vi "Begin.vi"(8 "error in (no error)":errorcluster, 11 "Two Drivers in":refnum<class "Two Drivers.lvclass">) -> (0 "error out":errorcluster, 3 "Two Drivers out":refnum<class "Two Drivers.lvclass">)   [LabVIEW 2018, in "Joysticks.lvlib" / "Two Drivers.lvclass"]
doc: "This VI is used to open the joystick control references."
uses:
  Two Drivers.lvclass
  <vilib>/Rock Robotics/WPI/Joystick/WPI_JoystickDeviceEnum.ctl
  Two Drivers.lvclass/Two Drivers.ctl
  Joysticks.lvclass
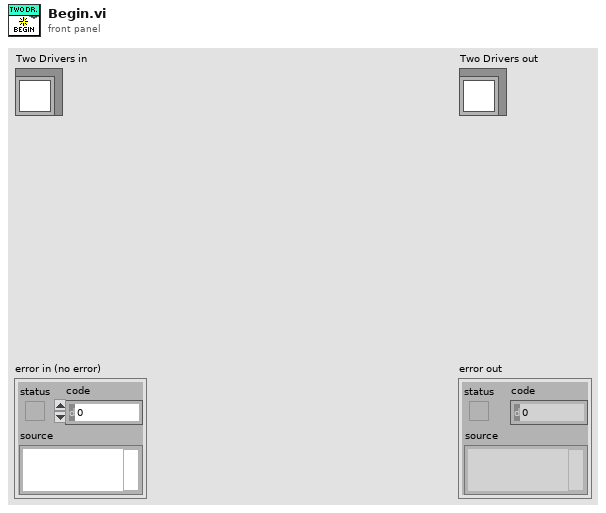
[diagram p1: front panel]
types:
  T1 = typedef "WPI_JoystickDeviceEnum.ctl" = enum16{"USB 0", "USB 1", "USB 2", "USB 3", "USB 4", "USB 5"}
  T2 = typedef "WPI_JoystickDevRef.ctl" = cluster{"Device":T1}
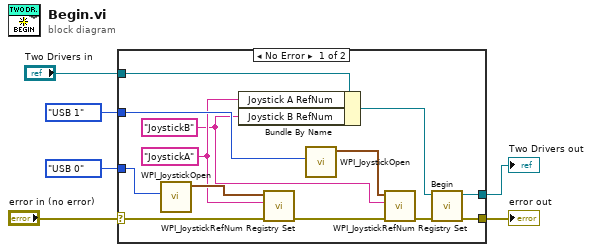
[diagram p0: block diagram]
diagram:
  n1 = case shown="No Error" "error in (no error)" {
    selector: "error in (no error)" -> [w14 w21]
    tunnel: [w19 w21] -> w2
    tunnel: [w18 w20] -> w3
    tunnel: "Two Drivers in" -> [w17 w20]
    tunnel: WPI_JoystickDeviceEnum."USB 0" ("JoystickDevice") -> [w11 _]
    tunnel: WPI_JoystickDeviceEnum."USB 1" ("JoystickDevice") -> [w10 _]
    frame No Error {
      w7 = "JoystickB" ("Joystick B RefNum")
      w8 = "JoystickA" ("Joystick A RefNum")
      n2 = call <vilib>:"WPI_JoystickOpen.vi"("JoystickDevice"=w11) -> ("JoystickDevRef"=w15:T2)  [unwired: 10 in]
      n3 = Bundle By Name(cluster=w17, "Joystick A RefNum"=w8, "Joystick B RefNum"=w7) -> (w9:refnum<class "Two Drivers.lvclass">)
      n4 = call <vilib>:"WPI_JoystickRefNum Registry Set.vi"("error in (no error)"=w14, "refnum name"=w8, "JoystickDevRef"=w15) -> ("error out"=w13:errorcluster)  [unwired: 7 in, 1 out]
      n5 = call <vilib>:"WPI_JoystickOpen.vi"("JoystickDevice"=w10) -> ("JoystickDevRef"=w16:T2)  [unwired: 10 in]
      n6 = call <vilib>:"WPI_JoystickRefNum Registry Set.vi"("error in (no error)"=w13, "refnum name"=w7, "JoystickDevRef"=w16) -> ("error out"=w12:errorcluster)  [unwired: 7 in, 1 out]
      n7 = call-parent "Begin.vi"("error in (no error)"=w12, "Joysticks in"=w9) -> ("error out"=w19:errorcluster, "Joysticks out"=w18:refnum<class "Two Drivers.lvclass">)  [unwired: 8 in]
    }
    frame Error {
    }
  }
  "error out" <- w2
  "Two Drivers out" <- w3
